vi "HDF5_Write_TC_alarm_record.vi"(4 "date/time string":string, 6 "current time":timestamp, 8 "error in":errorcluster, 10 "TC Alarms":T1, 11 "TCRef":T2 {"Alarm_Source_dset" format="%.0x"; "Time_AlarmChange_dset" format="%.0x"; "Time_Valid_dset" format="%.0x"; "Alarm_Valid_dset" format="%.0x"; "Saturat_dset" format="%.0x"; "Group_ref" format="%.0x"; "Weath_Valid_dset" format="%.0x"; "Disdr_Valid_dset" format="%.0x"}) -> (0 "error out":errorcluster)   [LabVIEW 2018]
doc: "Write a single Tone<x> record with timestamp:\nTone1\n Beac - cluster\n BeacZoom - 1024 element Double array (waveform) \n Cal - cluster\n CalZoom - 1024 element Double array (waveform)"
uses:
  HDF5_Validty_refs.ctl
  <vilib>/addons/h5labview2/base/hid_t.ctl
  TC_Data_Structure.ctl
  <vilib>/addons/h5labview2/base/lib_path.vi
  <vilib>/addons/h5labview2/base/H5Equery.vi
  <vilib>/addons/h5labview2/dataset/H5Dwrite.llb/H5Dwrite.xnode
  <vilib>/addons/h5labview2/dataset/H5D.lvlib
  <vilib>/addons/h5labview2/space/H5S.lvlib
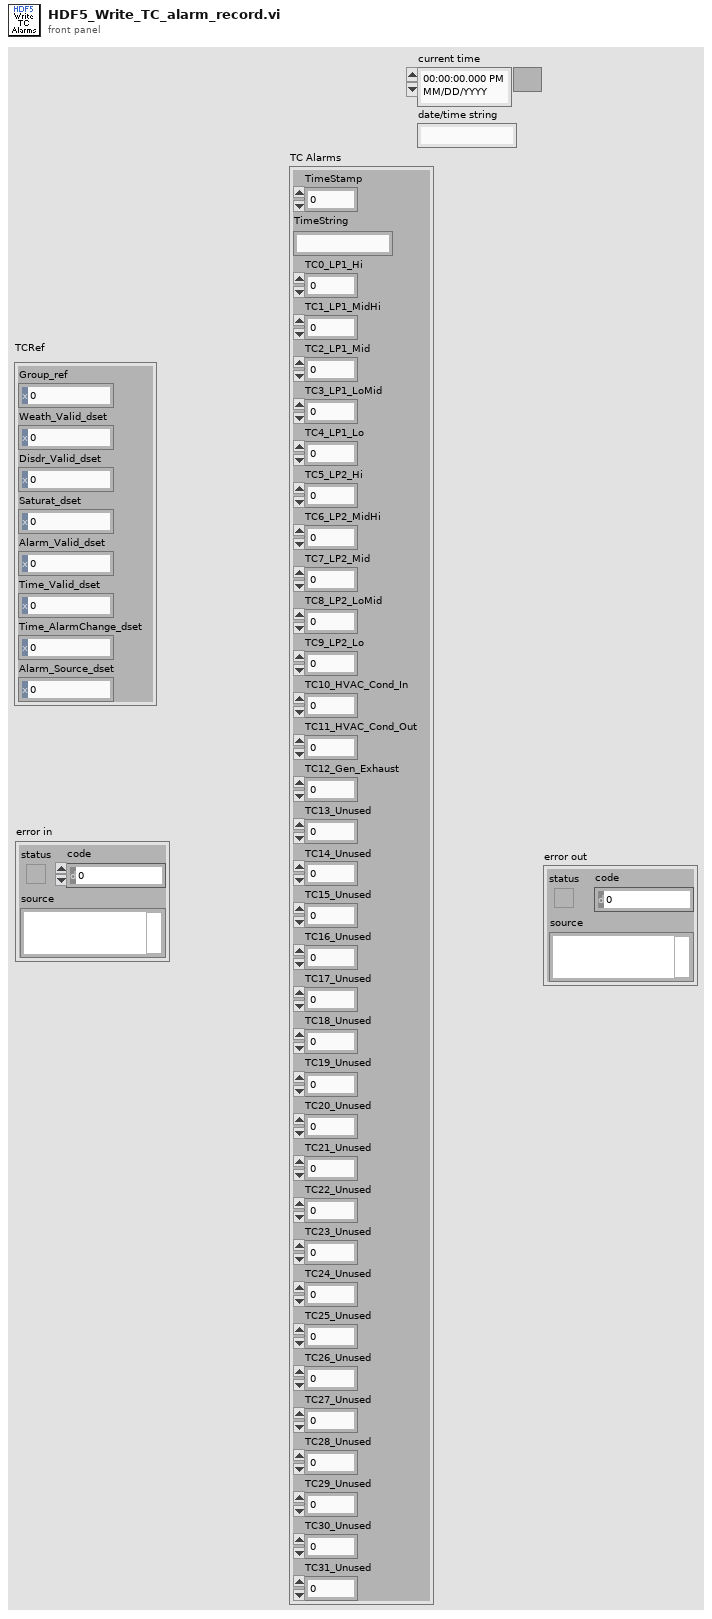
[diagram p1: front panel]
types:
  T1 = typedef "TC_Data_Structure.ctl" = cluster{"TimeStamp":dbl, "TimeString":string, "TC0_LP1_Hi":dbl, "TC1_LP1_MidHi":dbl, "TC2_LP1_Mid":dbl, "TC3_LP1_LoMid":dbl, "TC4_LP1_Lo":dbl, "TC5_LP2_Hi":dbl, "TC6_LP2_MidHi":dbl, "TC7_LP2_Mid":dbl, "TC8_LP2_LoMid":dbl, "TC9_LP2_Lo":dbl, "TC10_HVAC_Cond_In":dbl, "TC11_HVAC_Cond_Out":dbl, "TC12_Gen_Exhaust":dbl, "TC13_Unused":dbl, "TC14_Unused":dbl, "TC15_Unused":dbl, "TC16_Unused":dbl, "TC17_Unused":dbl, "TC18_Unused":dbl, "TC19_Unused":dbl, "TC20_Unused":dbl, "TC21_Unused":dbl, "TC22_Unused":dbl, "TC23_Unused":dbl, "TC24_Unused":dbl, "TC25_Unused":dbl, "TC26_Unused":dbl, "TC27_Unused":dbl, "TC28_Unused":dbl, "TC29_Unused":dbl, "TC30_Unused":dbl, "TC31_Unused":dbl}
  T2 = typedef "HDF5_Validty_refs.ctl" = cluster{"Group_ref":T3, "Weath_Valid_dset":T3, "Disdr_Valid_dset":T3, "Saturat_dset":T3, "Alarm_Valid_dset":T3, "Time_Valid_dset":T3, "Time_AlarmChange_dset":T3, "Alarm_Source_dset":T3}
  T3 = typedef "hid_t.ctl" = i32
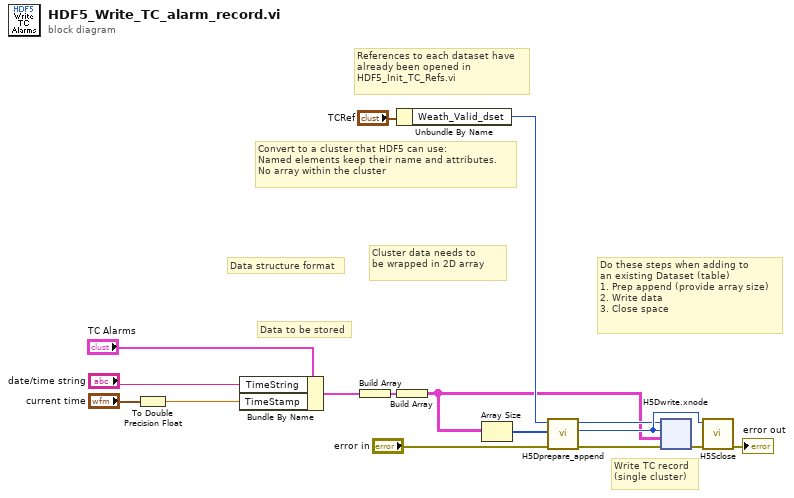
[diagram p0: block diagram]
diagram:
  # "Convert to a cluster that HDF5 can use:\nNamed elements keep their name and attributes.\nNo array within the cluster"
  # "Cluster data needs to \nbe wrapped in 2D array"
  # "Data to be stored"
  # "Data structure format"
  # "References to each dataset have \nalready been opened in \nHDF5_Init_TC_Refs.vi"
  # "Do these steps when adding to \nan existing Dataset (table)\n1. Prep append (provide array size)\n2. Write data\n3. Close space"
  # "Write TC record\n(single cluster)"
  n1 = To Double Precision Float(number="current time") -> (double precision float=w2:dbl)
  n2 = Bundle By Name(cluster="TC Alarms", "TimeString"="date/time string", "TimeStamp"=w2) -> (w8:T1)
  n3 = Build Array(w8) -> (w7:T1[])
  n4 = Unbundle By Name("TCRef") -> ("Weath_Valid_dset"=w10:T3)
  n5 = Build Array(w7) -> (w6:T1[][])
  n6 = Array Size(array=w6) -> (size(s)=w5:i32[])
  n7 = call <vilib>:"H5Dprepare_append.vi"("error in (no error)"="error in", "append dims"=w5, "dset in"=w10) -> ("error out"=w16:errorcluster, "space out"=w14:T3, "dset out"=w13:T3)  [unwired: 5 in, 1 out]
  n8 = xnode "H5Dwrite.xnode"("error in (no error)"=w16, "data"=w6, "file space"=w14, "ref in"=w13) -> ("error out"=w15:errorcluster)  [unwired: 3 in, 2 out]
  n9 = call <vilib>:"H5Sclose.vi"("error in (no error)"=w15, "space in"=w14) -> ("error out"=→"error out":errorcluster)  [unwired: 9 in]
